vi "sub_picture_gnss-deg.vi"(8 "pen":T1={"Width"=1, "Style"=enum."Solid"}, 9 "radius":i16=64, 10 "Center":dbl=80.0 format="%#_13g", 11 "deg_gps":dbl) -> (3 "new picture":picture)   [LabVIEW 2019]
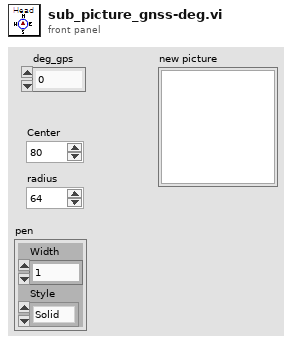
[diagram p1: front panel]
types:
  T1 = cluster{"Width":u16, "Style":enum32{"Solid", "Dash", "Dot", "DashDot", "DashDotDot"}}
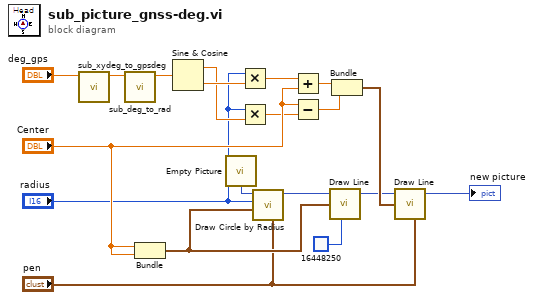
[diagram p0: block diagram]
diagram:
  n1 = call "sub_xydeg_to_gpsdeg.vi"("xy deg in"="deg_gps") -> ("gps deg out"=w17:dbl)  [unwired: 10 in]
  n2 = call "sub_deg_to_rad.vi"("deg in"=w17) -> ("rad out"=w4:dbl)  [unwired: 10 in]
  n3 = Bundle("Center"="Center", "Center"="Center") -> (w19:cluster{"Center":dbl, "Center":dbl})  [unwired: 1 in]
  n4 = Sine & Cosine(0:w4) -> (1:w2:dbl, 2:w3:dbl)
  n5 = call "Empty Picture"() -> ("empty picture"=w5:picture)
  n6 = Multiply(x="radius", y=w3) -> (x*y=w11:dbl)
  n7 = Multiply(x="radius", y=w2) -> (x*y=w14:dbl)
  n8 = call <vilib>:"Draw Circle by Radius.vi"("pen"="pen", "pixel center"=w19, "radius"="radius", "picture"=w5) -> ("new picture"=w6:picture)  [unwired: 7 in]
  n9 = Add(x=w11, y="Center") -> (x+y=w12:dbl)
  n10 = Subtract(x="Center", y=w14) -> (x-y=w15:dbl)
  n11 = call <vilib>:"Draw Line.vi"("picture"=w6, "end point"=w19, "color(black)"=u32 16448250) -> ("new picture"=w7:picture)  [unwired: 6 in]
  n12 = Bundle(w12, w15) -> (w13:cluster{dbl, dbl})  [unwired: 1 in]
  n13 = call <vilib>:"Draw Line.vi"("picture"=w7, "end point"=w13, "pen"="pen") -> ("new picture"=→"new picture":picture)  [unwired: 6 in]
